vi "Executor.vi"(8 "error in (no error)":errorcluster caption="错误输入（无错误）", 10 "WriteBuff":string, 11 "Serial 输入":refnum<class "Serial.lvclass"> caption="DNL_LabVIEW Object in") -> (0 "error out":errorcluster caption="错误输出", 1 "ReadLength":i32, 2 "ReadBuf":string, 3 "Serial 输出":refnum<class "Serial.lvclass"> caption="DNL_LabVIEW Object out")   [LabVIEW 2012, in "Serial.lvclass"]
uses:
  Serial.lvclass
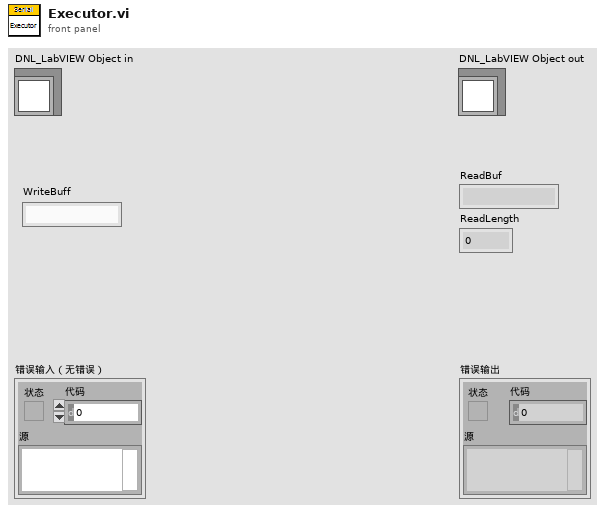
[diagram p1: front panel]
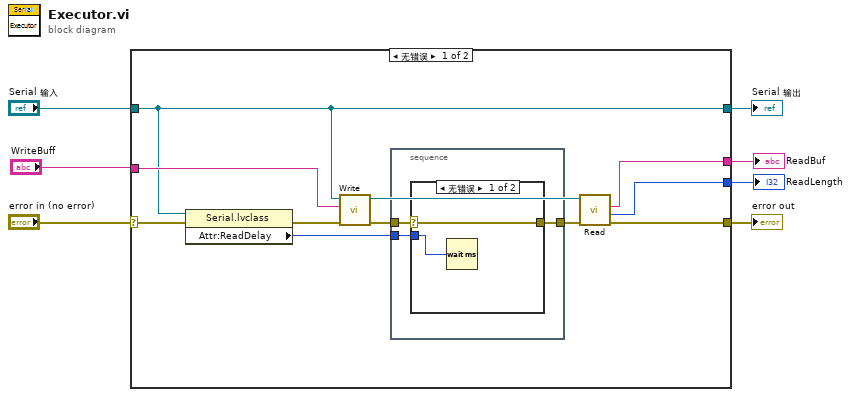
[diagram p0: block diagram]
diagram:
  n1 = case shown="无错误" "error in (no error)" {
    selector: "error in (no error)" -> [w18 w26]
    tunnel: [w10 w26] -> w6
    tunnel: [w15 w25] -> w4
    tunnel: "Serial 输入" -> [w15 w25]
    tunnel: "WriteBuff" -> [w16 _]
    tunnel: [w9 _] -> w2
    tunnel: [w8 _] -> w1
    frame No Error {
      n2 = property class="Serial.lvclass"(reference=w15, error in=w18) -> (error out=w17:errorcluster, "Attr:ReadDelay"=w13:u32)  [unwired: 1 out]
      n3 = call-dynamic "Write.vi"("error in (no error)"=w17, "buf"=w16, "Serial 输入"=w15) -> ("error out"=w14:errorcluster, "Serial 输出"=w11:refnum<class "Serial.lvclass">)  [unwired: 7 in]
      n4 = stacked-sequence {
        tunnel: w14 -> [w21]
        tunnel: w13 -> [w20]
        tunnel: [w19] -> w12
        frame #0 {
          n5 = case shown="无错误" w21 {
            selector: w21 -> [w22 w24]
            tunnel: w20 -> [w23 _]
            tunnel: [w22 w24] -> w19
            frame No Error {
              n6 = Wait (ms)(milliseconds to wait=w23) -> ()  [unwired: 1 out]
            }
            frame Error {
            }
          }
        }
      }
      n7 = call-dynamic "Read.vi"("error in (no error)"=w12, "Serial 输入"=w11) -> ("error out"=w10:errorcluster, "ReadLength"=w8:i32, "ReadBuf"=w9:string)  [unwired: 6 in, 1 out]
    }
    frame Error {
    }
  }
  "error out" <- w6
  "Serial 输出" <- w4
  "ReadBuf" <- w2
  "ReadLength" <- w1
